vi "timer.vi"(8 "error in (no error)":errorcluster, 9 "action":T1=enum."timeElapsed", 10 "Time to elapse latch":dbl, 11 "Time to elapse (s)":dbl) -> (0 "error out":errorcluster, 1 "time elapsed latch":bool, 2 "timeElapsed?":bool, 3 "Time":dbl)   [LabVIEW 2024]
doc: "Sends TRUE if time elapsed [Time to elapse (s)]. 'Time to elapse latch' sets time to switch between TRUE and FALSE."
uses:
  Controls/#typedef_action_timer.ctl
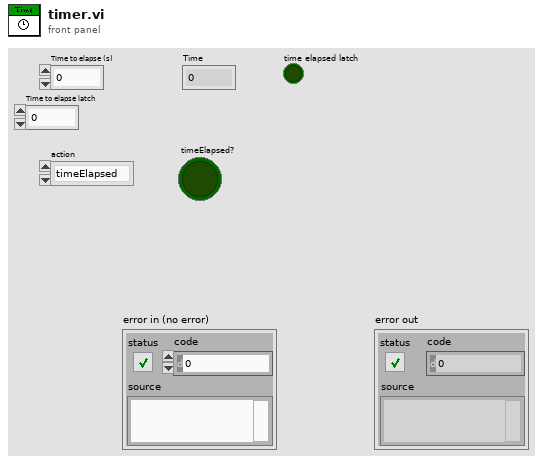
[diagram p1: front panel]
types:
  T1 = typedef "#typedef_action_timer.ctl" = enum16{"reset", "timeElapsed"}
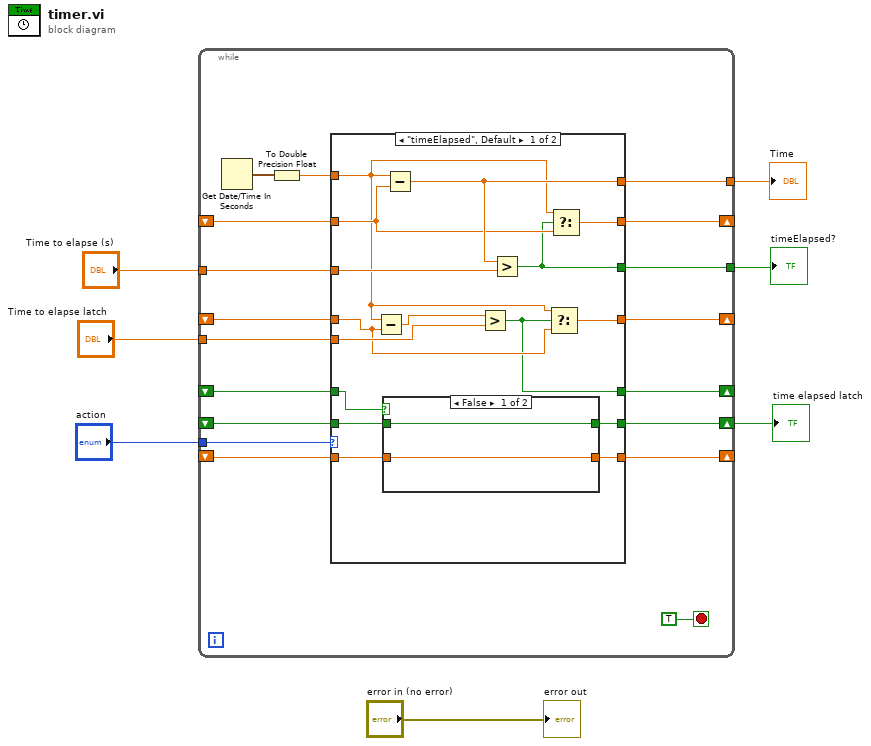
[diagram p0: block diagram]
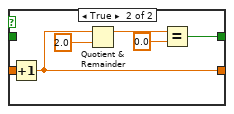
[diagram p2: hidden frame]
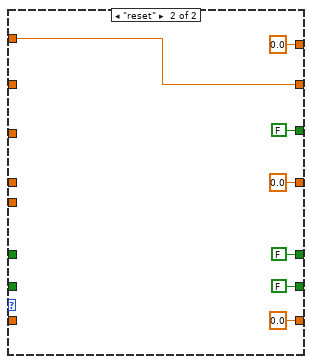
[diagram p3: hidden frame]
diagram:
  n1 = while {
    shift-right: [w20] -> _
    shift-left: _ -> [w22]
    tunnel: "action" -> [w24]
    tunnel: [w21] -> w6
    tunnel: "Time to elapse (s)" -> [w19]
    tunnel: [w17] -> w7
    shift-right: [w8] -> _
    shift-left: _ -> [w16]
    shift-right: [w13] -> _
    shift-left: _ -> [w14]
    shift-right: [w15] -> w2
    shift-left: _ -> [w12]
    tunnel: "Time to elapse latch" -> [w11]
    shift-right: [w10] -> _
    shift-left: _ -> [w9]
    stop <- TRUE stop-if-true
    n2 = Get Date/Time In Seconds() -> (seconds since 1Jan1904=w25:timestamp)
    n3 = To Double Precision Float(number=w25) -> (double precision float=w23:dbl)
    n4 = case shown="\"timeElapsed\", Default" w24 {
      tunnel: w23 -> [w29 w56]
      tunnel: w22 -> [w39 _]
      tunnel: [w40 0.0] -> w21
      tunnel: [w41 w56] -> w20
      tunnel: w19 -> [w38 _]
      tunnel: [w37 FALSE] -> w17
      tunnel: w16 -> [w34 _]
      tunnel: [w33 FALSE] -> w15
      tunnel: w14 -> [w36 _]
      tunnel: [w35 0.0] -> w13
      tunnel: w12 -> [w32 _]
      tunnel: w11 -> [w31 _]
      tunnel: [w30 0.0] -> w10
      tunnel: w9 -> [w27 _]
      tunnel: [w26 FALSE] -> w8
      frame "timeElapsed", Default {
        n5 = Subtract(x=w29, y=w27) -> (x-y=w28:dbl)
        n6 = case shown="False" w34 {
          tunnel: w36 -> [w43 w49]
          tunnel: [w43 w48] -> w35
          tunnel: [w42 w44] -> w33
          tunnel: w32 -> [w42 _]
          frame False {
          }
          frame True {
            n7 = Increment(x=w49) -> (x+1=w48:dbl)
            n8 = Quotient & Remainder(x=w48, y=2.0) -> (x-y*floor(x/y)=w46:dbl)  [unwired: 1 out]
            n9 = Equal?(x=w46, y=0.0) -> (x = y?=w44:bool)
          }
        }
        n10 = Subtract(x=w29, y=w39) -> (x-y=w40:dbl)
        n11 = Greater?(x=w28, y=w31) -> (0:w26:bool)
        n12 = Greater?(x=w40, y=w38) -> (0:w37:bool)
        n13 = Select(t=w29, s=w26, f=w27) -> (s? t:f=w30:dbl)
        n14 = Select(t=w29, s=w37, f=w39) -> (s? t:f=w41:dbl)
      }
      frame "reset" {
      }
    }
  }
  "timeElapsed?" <- w7
  "Time" <- w6
  "time elapsed latch" <- w2
  "error out" <- "error in (no error)"
